vi "nelder_best_worst.vi"(8 "error in":errorcluster, 11 "array":sgl[][](array[numeric])) -> (0 "error out":errorcluster, 1 "worst":sgl, 2 "second worst":sgl, 3 "best":sgl)   [LabVIEW 2018]
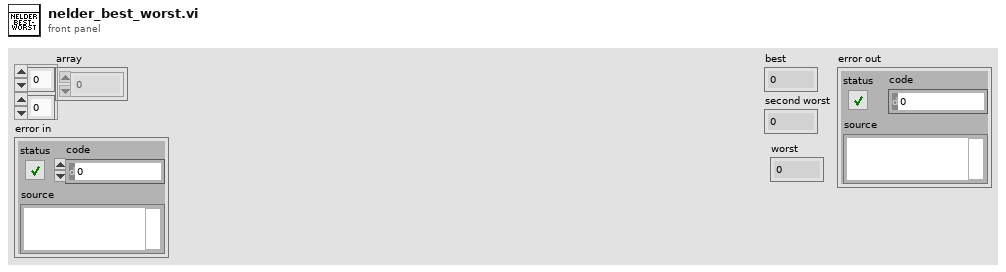
[diagram p1: front panel]
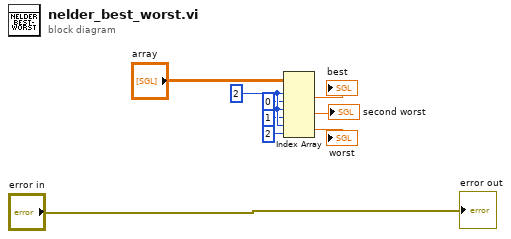
[diagram p0: block diagram]
diagram:
  w8 = 2 ("index (row)")
  n1 = Index Array(array="array", index (row) #1=w8, index (col) #1=0 ("disabled index (col)"), index (row) #2=w8, index (col) #2=1 ("disabled index (col)"), index (row) #3=w8, index (col) #3=2 ("disabled index (col)")) -> (element #1=→"best":sgl, element #2=→"second worst":sgl, element #3=→"worst":sgl)
  "error out" <- "error in"
